vi "Listen for Claim.vi"(0 "session in":refnum<k21>, 5 "ref in":T1, 7 "Requested Addresses":u8[](array[numeric]), 9 "timeout (0)":dbl, 11 "error in":errorcluster) -> (4 "session out":refnum<k21>, 6 "Conflict?":bool, 8 "Conflict Indeces":i32[](array[numeric]), 15 "error out":errorcluster)   [LabVIEW 2015, in "J1939 Addon Engine.lvlib"]
uses:
  J1939 Addon Engine.lvlib
  Types/Address Table Reference.ctl
  Types/Address Lookup Table Action.ctl
  Shared/Types/Address Lookup Table Data.ctl
  Shared/J1939 Utilities/SubVIs/Convert CAN Arb ID to J1939 ID.vi
  Address Lookup Table.vi
  <vilib>/xnet/xnet.llb/XNET Read (Frame CAN).vi
  Shared/J1939 Utilities/J1939 Utilities.lvlib
  Shared/J1939 Addon Shared.lvlib
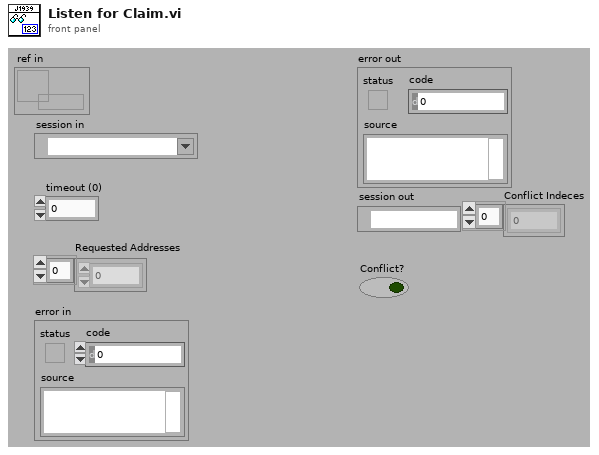
[diagram p1: front panel]
types:
  T1 = typedef "J1939 Addon Engine.lvlib/Address Table Reference.ctl" = refnum<data-value>
  T2 = typedef "J1939 Addon Shared.lvlib/Address Lookup Table Data.ctl" = cluster{"Name":u8[], "Address":u8}
  T3 = typedef "J1939 Addon Engine.lvlib/Address Lookup Table Action.ctl" = enum16{"Initialize", "Add", "Get", "Remove", "Get All"}
  T4 = typedef "XNET Frame CAN.ctl" = cluster{"timestamp":timestamp, "payload":u8[], "identifier":u32, "type":T5, "extended?":bool, "echo?":bool}
  T5 = typedef "XNET Frame Type CAN.ctl" = u8
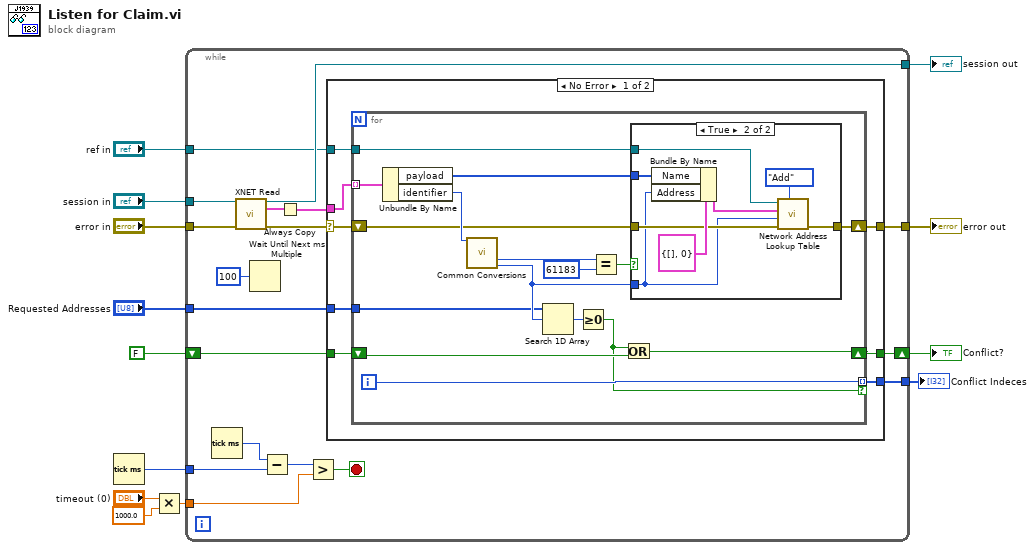
[diagram p0: block diagram]
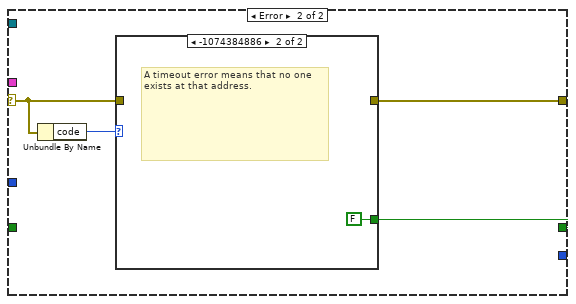
[diagram p3: hidden frame]
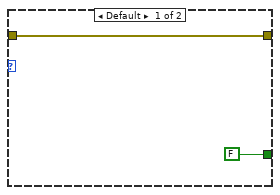
[diagram p4: hidden frame]
diagram:
  n1 = Tick Count (ms)() -> (millisecond timer value=w6:u32)
  n2 = Multiply(x="timeout (0)", y=1000.0) -> (x*y=w3:dbl)
  n3 = while {
    tunnel: "session in" -> [w31]
    tunnel: "Requested Addresses" -> [w30]
    tunnel: w3 -> [w17]
    tunnel: "error in" -> [w26]
    tunnel: [w25] -> w10
    tunnel: [w24] -> w9
    shift-right: [w28] -> w12
    shift-left: FALSE -> [w23]
    tunnel: "ref in" -> [w22]
    tunnel: w6 -> [w19]
    tunnel: [w14] -> w1
    stop <- w16 stop-if-true
    n4 = Tick Count (ms)() -> (millisecond timer value=w20:u32)
    n5 = call-poly <vilib>:"XNET Read.vi"("session in"=w31, "error in (no error)"=w26) -> ("session out"=w24:refnum<k21>, "data"=w27:T4[], "error out"=w29:errorcluster)  [unwired: 11 out]
    n6 = Wait Until Next ms Multiple(millisecond multiple=u32 100) -> ()  [unwired: 1 out]
    n7 = Subtract(x=w20, y=w19) -> (x-y=w18:u32)
    n8 = Always Copy(1:w27) -> (0:w15:T4[])
    n9 = Greater?(x=w18, y=w17) -> (0:w16:bool)
    n10 = case shown="No Error" w29 {
      selector: w29 -> [w35 w65]
      tunnel: w30 -> [w39 _]
      tunnel: w15 -> [w38 _]
      tunnel: [w37 w67] -> w28
      tunnel: [w34 w66] -> w25
      tunnel: w23 -> [w36 _]
      tunnel: w22 -> [w33 _]
      tunnel: [w32 _] -> w14
      frame No Error {
        n11 = for {
          tunnel: w38 -> [w55] mode=indexing
          tunnel: w39 -> [w43]
          shift-right: [w41] -> w37
          shift-left: w36 -> [w47]
          shift-right: [w45] -> w34
          shift-left: w35 -> [w46]
          tunnel: w33 -> [w44]
          tunnel: [w42] -> w32 mode=indexing if=w40
          i -> [w42]
          n12 = Unbundle By Name(w55) -> ("payload"=w49:u8[], "identifier"=w54:u32)
          n13 = call-poly "Common Conversions.vi"("Arb ID"=w54) -> ("PGN"=w53:u32, "Source Address"=w50:u8)  [unwired: 11 in, 2 out]
          n14 = Search 1D Array(1D array=w43, element=w50) -> (index of element=w48:i32)  [unwired: 1 in]
          n15 = Greater Or Equal To 0?(x=w48) -> (x >= 0?=w40:bool)
          n16 = Equal?(x=w53, y=u32 61183) -> (x = y?=w51:bool)
          n17 = Or(x=w40, y=w47) -> (x .or. y?=w41:bool)
          n18 = case shown="True" w51 {
            tunnel: w50 -> [_ w57]
            tunnel: w49 -> [_ w63]
            tunnel: w46 -> [w56 w60]
            tunnel: [w56 w59] -> w45
            tunnel: w44 -> [_ w58]
            frame False {
            }
            frame True {
              n19 = Bundle By Name(cluster=T2 {"Name"=[], "Address"=0} ("Data"), "Name"=w63, "Address"=w57) -> (w61:T2)
              n20 = call "Network Address Lookup Table.vi"("Action"=Address_Lookup_Table_Action."Add", "error in (no error)"=w60, "Address"=w57, "Data"=w61, "Address LUT"=w58) -> ("error out"=w59:errorcluster)  [unwired: 2 in, 4 out]
            }
          }
        }
      }
      frame Error {
        n21 = Unbundle By Name(w65) -> ("code"=w68:i32)
        n22 = case shown="-1074384886" w68 {
          tunnel: [FALSE FALSE] -> w67
          tunnel: [w69 _] -> w66
          tunnel: w65 -> [w69 _]
          frame Default {
          }
          frame -1074384886 {
            # "A timeout error means that no one exists at that address."
          }
        }
      }
    }
  }
  "Conflict?" <- w12
  "error out" <- w10
  "session out" <- w9
  "Conflict Indeces" <- w1
